vi "Find Analog Replay.vi"(8 "error in (no error)":errorcluster, 10 "Name":string, 11 "APU Node in":refnum<k24>) -> (0 "error out":errorcluster, 2 "Analog Replay out":refnum<k24>, 3 "APU Node out":refnum<k24>)   [LabVIEW 2015, in "Engine Simulation Toolkit SysDef API.lvlib"]
uses:
  Engine Simulation Toolkit SysDef API.lvlib
  NationalInstruments.VeriStand.SystemDefinitionAPI
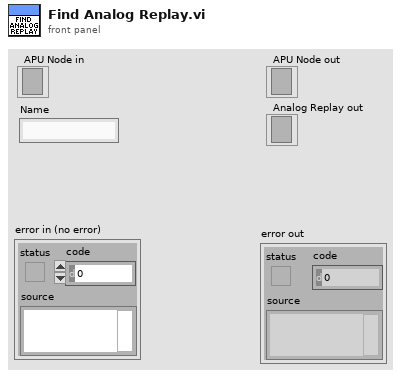
[diagram p1: front panel]
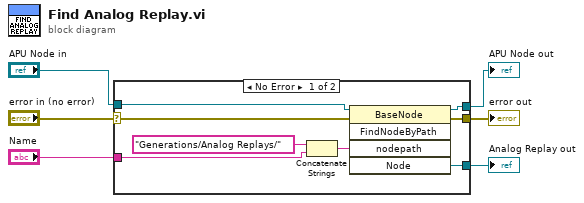
[diagram p0: block diagram]
diagram:
  n1 = case shown="No Error" "error in (no error)" {
    selector: "error in (no error)" -> [w7 w16]
    tunnel: [w9 w16] -> w6
    tunnel: "APU Node in" -> [w11 w15]
    tunnel: [w10 w15] -> w3
    tunnel: [w8 _] -> w2
    tunnel: "Name" -> [w13 _]
    frame No Error {
      n2 = Concatenate Strings("Generations/Analog Replays/" ("nodepath"), w13) -> (w12:string)
      n3 = invoke class="BaseNode" method="FindNodeByPath"(reference=w11, error in=w7, "nodepath"=w12) -> (reference out=w10:refnum<k24>, error out=w9:errorcluster, "Node"=w8:refnum<k24>)  [unwired: 2 in, 2 out]
    }
    frame Error {
    }
  }
  "error out" <- w6
  "Analog Replay out" <- w2
  "APU Node out" <- w3
